vi "inteference -- find center V2.vi"(7 "number of points":i32, 8 "complex region":T1={"max re"=5.161869466666667e-06, "min re"=5.176843333333334e-06, "max im"=-2.467216e-05, "min im"=-0.001573233, "delta re"=0.003211203, "delta im"=0.00165815, "center re"=0.0015485608400000002, "delta  z"=0.0015530530000000002+0.0i, "center im"=0.0, "center z"=0.0+0.0i, "d im"=0.0, "d re"=0.0, "d z"=0.0+0.0i}, 9 "pond":cdb[][](array[numeric]), 10 "point sources":cdb[](array[numeric]), 11 "wave packet":cdb[][](array[numeric])) -> (2 "z (center)":cdb)   [LabVIEW 2018]
uses:
  complex region.ctl
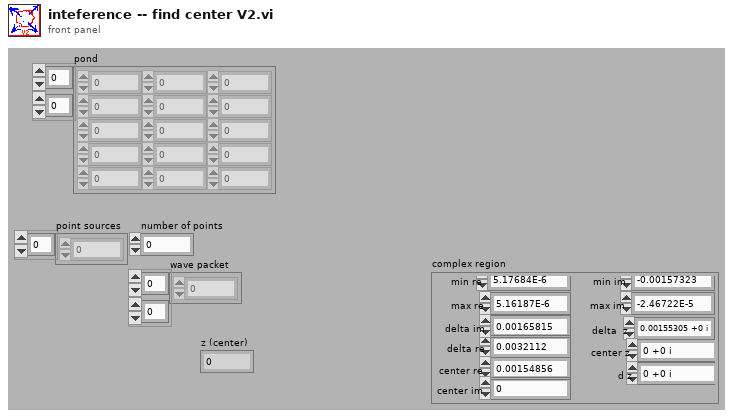
[diagram p1: front panel]
types:
  T1 = typedef "complex region.ctl" = cluster{"max re":dbl, "min re":dbl, "max im":dbl, "min im":dbl, "delta re":dbl, "delta im":dbl, "center re":dbl, "delta  z":cdb, "center im":dbl, "center z":cdb, "d im":dbl, "d re":dbl, "d z":cdb}
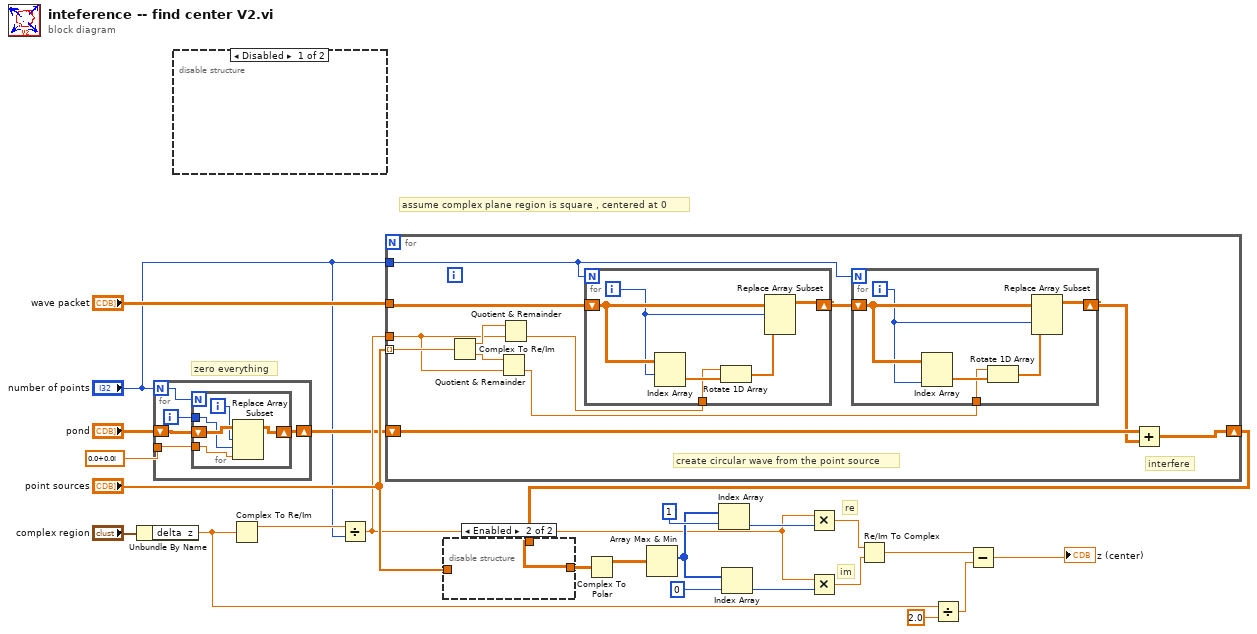
[diagram p0: block diagram]
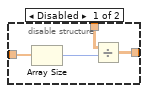
[diagram p3: hidden frame]
diagram:
  # "zero everything"
  # "assume complex plane region is square , centered at 0"
  # "re"
  # "im"
  n1 = Unbundle By Name("complex region") -> ("delta  z"=w9:cdb)
  n2 = for {
    N: "number of points" -> [w25]
    tunnel: cdb 0.0+0.0i -> [w28]
    shift-right: [w26] -> w4
    shift-left: "pond" -> [w29]
    i -> [w27]
    n3 = for {
      N: w25 -> [_]
      tunnel: w28 -> [w30]
      tunnel: w27 -> [w33]
      shift-right: [w32] -> w26
      shift-left: w29 -> [w34]
      i -> [w31]
      n4 = Replace Array Subset(array=w34, new element=w30, index (row)=w31, index (col)=w33) -> (w32:cdb[][])
    }
  }
  n5 = disable-structure shown="Disabled" {
    frame Disabled {
    }
    frame Enabled {
    }
  }
  n6 = Complex To Re/Im(x + iy=w9) -> (x=w13:dbl)  [unwired: 1 out]
  n7 = Divide(x=w13, y="number of points") -> (x/y=w5:dbl)
  n8 = for {
    shift-right: [w45] -> w24
    shift-left: w4 -> [w46]
    tunnel: "point sources" -> [w36] mode=indexing
    tunnel: "wave packet" -> [w39]
    tunnel: w5 -> [w35]
    tunnel: "number of points" -> [w41]
    # "interfere"
    # "create circular wave from the point source"
    n9 = Complex To Re/Im(x + iy=w36) -> (x=w44:dbl, y=w43:dbl)
    n10 = Quotient & Remainder(x=w43, y=w35) -> (floor(x/y)=w37:dbl)  [unwired: 1 out]
    n11 = Quotient & Remainder(x=w44, y=w35) -> (floor(x/y)=w38:dbl)  [unwired: 1 out]
    n12 = for {
      N: w41 -> [_]
      shift-right: [w58] -> w42
      shift-left: w39 -> [w57]
      tunnel: w38 -> [w54]
      i -> [w53]
      n13 = Index Array(array=w57, index (row)=w53) -> (element=w55:cdb[])  [unwired: 1 in]
      n14 = Rotate 1D Array(1:w55, 2:w54) -> (0:w56:cdb[])
      n15 = Replace Array Subset(array=w57, new element=w56, index (row)=w53) -> (w58:cdb[][])  [unwired: 1 in]
    }
    n16 = for {
      N: w41 -> [_]
      shift-right: [w52] -> w40
      shift-left: w42 -> [w51]
      tunnel: w37 -> [w48]
      i -> [w47]
      n17 = Index Array(array=w51, index (col)=w47) -> (element=w49:cdb[])  [unwired: 1 in]
      n18 = Rotate 1D Array(1:w49, 2:w48) -> (0:w50:cdb[])
      n19 = Replace Array Subset(array=w51, new element=w50, index (col)=w47) -> (w52:cdb[][])  [unwired: 1 in]
    }
    n20 = Add(x=w46, y=w40) -> (x+y=w45:cdb[][])
  }
  n21 = disable-structure shown="Enabled" {
    disable-tunnel: w24 -> [w62 w63]
    disable-tunnel: "point sources" -> [w60 _]
    disable-tunnel: [w59 w63] -> w18
    frame Disabled {
      n22 = Array Size(array=w60) -> (size(s)=w61:i32)
      n23 = Divide(x=w62, y=w61) -> (x/y=w59:cdb[][])
    }
    frame Enabled {
    }
  }
  n24 = Complex To Polar(r * e^(i*theta)=w18) -> (r=w17:dbl[][])  [unwired: 1 out]
  n25 = Array Max & Min(array=w17) -> (max index (indices)=w16:i32[])  [unwired: 3 out]
  n26 = Index Array(array=w16, index=1) -> (element=w15:i32)
  n27 = Index Array(array=w16, index=0) -> (element=w14:i32)
  n28 = Multiply(x=w5, y=w15) -> (x*y=w12:dbl)
  n29 = Multiply(x=w5, y=w14) -> (x*y=w11:dbl)
  n30 = Re/Im To Complex(1:w11, 2:w12) -> (0:w7:cdb)
  n31 = Divide(x=w9, y=2.0) -> (x/y=w8:cdb)
  n32 = Subtract(x=w7, y=w8) -> (x-y=→"z (center)":cdb)
